vi "Tmp_M simulated readout all.vi"(8 "error in (no error)":errorcluster, 11 "VISA Refnum in":refnum<visa-resource-name>) -> (0 "error out":errorcluster, 2 "LSC218 sensors":T1 {"Time stamp" format="%<%H:%M:%S%2u\n%Y/%m/%d>T"}, 3 "VISA Refnum out":refnum<visa-resource-name>)   [LabVIEW 2017, in "Magnet module.lvlib"]
doc: "Queries Temperature monitor (LSC218) for all values from sensors in cryostat."
uses:
  Magnet module.lvlib
  ctl/Cryostat temperature sensors.ctl
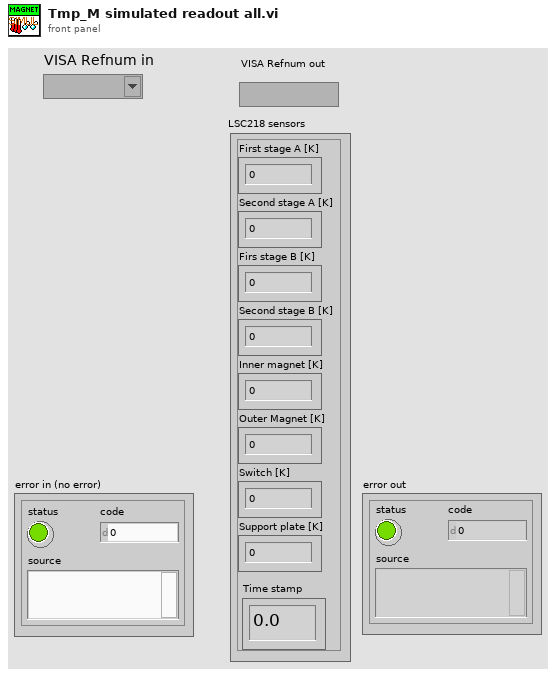
[diagram p1: front panel]
types:
  T1 = typedef "Magnet module.lvlib/Cryostat temperature sensors.ctl" = cluster{"First stage A [K]":dbl, "Second stage A [K]":dbl, "Firs stage B [K]":dbl, "Second stage B [K]":dbl, "Inner magnet [K]":dbl, "Outer Magnet [K]":dbl, "Switch [K]":dbl, "Support plate [K]":dbl, "Time stamp":dbl}
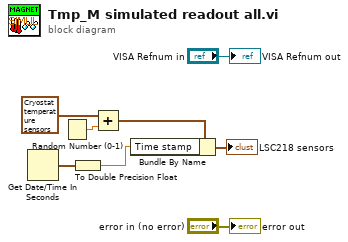
[diagram p0: block diagram]
diagram:
  n1 = Get Date/Time In Seconds() -> (seconds since 1Jan1904=w6:timestamp)
  n2 = Random Number (0-1)() -> (number: 0 to 1=w5:dbl)
  n3 = To Double Precision Float(number=w6) -> (double precision float=w2:dbl)
  n4 = Add(x=T1 {"First stage A [K]"=52.0, "Second stage A [K]"=9.0, "Firs stage B [K]"=51.0, "Second stage B [K]"=10.0, "Inner magnet [K]"=8.0, "Outer Magnet [K]"=7.0, "Switch [K]"=30.0, "Support plate [K]"=20.0, "Time stamp"=0.0} ("LSC218 sensors 2"), y=w5) -> (x+y=w4:T1)
  n5 = Bundle By Name(cluster=w4, "Time stamp"=w2) -> (→"LSC218 sensors":T1)
  "VISA Refnum out" <- "VISA Refnum in"
  "error out" <- "error in (no error)"
